vi "Actor Core.vi"(8 "error in":errorcluster, 11 "Fluke Hydra 2625A in":refnum<class "Fluke Hydra 2625A.lvclass">) -> (0 "error out":errorcluster, 3 "Actor out":refnum<class "Actor.lvclass">)   [LabVIEW 2014, in "Generic Data Acquisition.lvlib" / "Fluke Hydra.lvlib" / "Fluke Hydra 2625A.lvclass"]
doc: "(<B>Filename</B>: Actor Framework.lvlib:Actor.lvclass:Actor Core.vi)\n\nReceives messages to the actor, reacts to them, and initiates any error handling that may shut the actor down.\n\nDescendant classes may override this VI to append parallel tasks for the actor to complete while it handles messages. Overrides use the Call Parent Method node."
uses:
  Fluke Hydra 2625A.lvclass
  <vilib>/ActorFramework/Actor/Actor.lvclass
  <vilib>/ActorFramework/Actor/Actor.lvclass/Actor.ctl
  <vilib>/ActorFramework/Message Enqueuer/Message Enqueuer.lvclass/Message Enqueuer.ctl
  Display Panel/Display Panel V3 Messages/Write signal from control Msg/Write signal from control Msg.lvclass/Write signal from control Msg.ctl
  <vilib>/ActorFramework/Stop Msg/Stop Msg.lvclass/Stop Msg.ctl
  <vilib>/ActorFramework/Message Enqueuer/Init from Existing Queue.vi
  <vilib>/ActorFramework/Message Enqueuer/Enqueue.vi
  <vilib>/ActorFramework/Message Enqueuer/Enqueue Critical.vi
  <vilib>/ActorFramework/Message Priority Queue/Priority Enqueue.vi
  <vilib>/ActorFramework/Message Enqueuer/Message Enqueuer.lvclass
  Display Panel/Display Panel V3 Messages/Write signal from control Msg/Write signal from control Msg.lvclass
  Generic Data Acquisition Messages/Measure Msg/Measure Msg.lvclass
  <vilib>/ActorFramework/Stop Msg/Stop Msg.lvclass
  Generic Data Acquisition.lvclass
  Data Logger/Data Logger.lvclass
panel:
  out "i":i32
  out "Channel Names":string[](array[string])
  out "Channel Functions":i8[](array[numeric])
  out "Channel List":i8[](array[numeric])
  out "outside i":i32
  in  "Array":dbl[](array[numeric])=[0.0, 0.0]
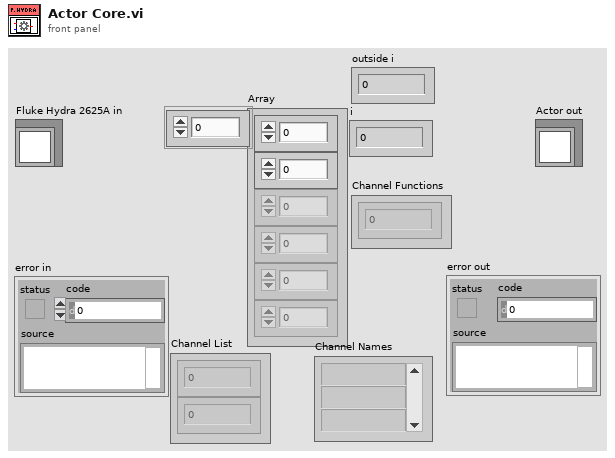
[diagram p1: front panel]
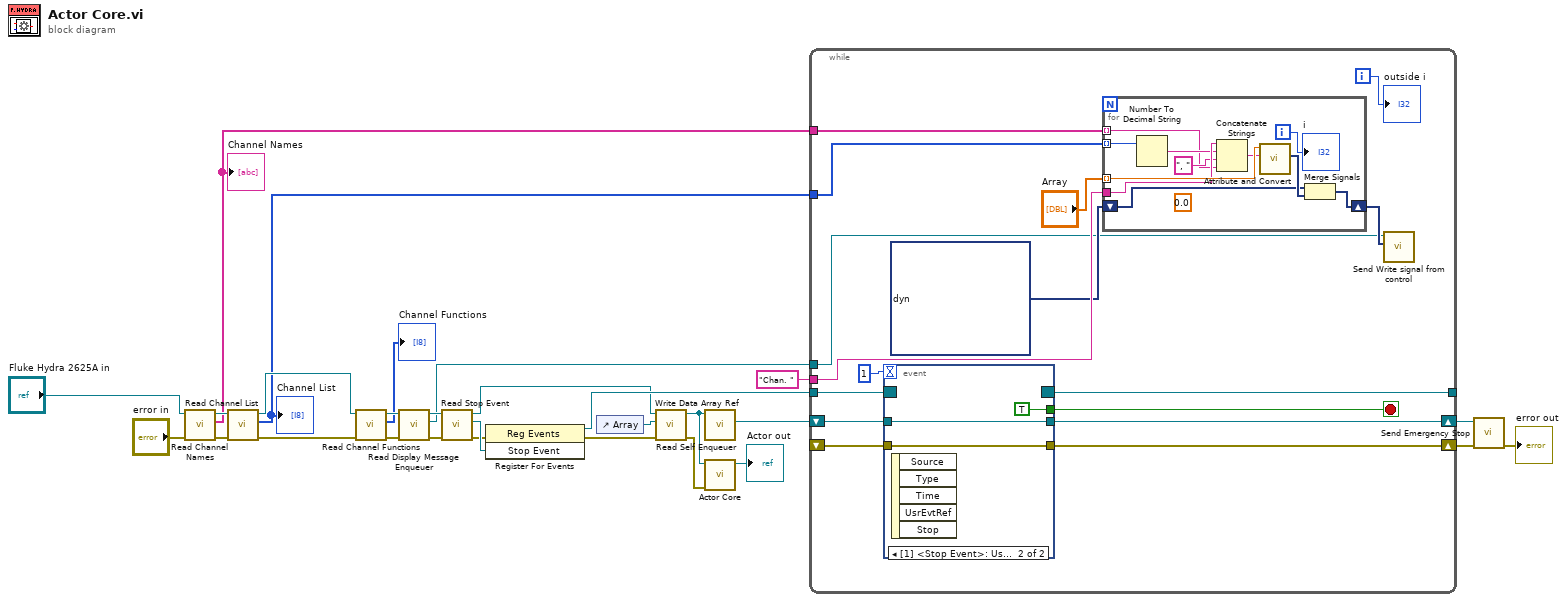
[diagram p0: block diagram]
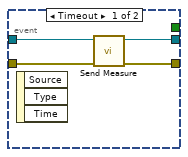
[diagram p2: hidden frame]
diagram:
  n1 = call-dynamic "Read Channel Names.vi"("error in (no error)"="error in", "Generic Data Acquisition in"="Fluke Hydra 2625A in") -> ("error out"=w4:errorcluster, "Channel Names"=w1:string[], "Generic Data Acquisition out"=w6:refnum<class "Fluke Hydra 2625A.lvclass">)  [unwired: 7 in]
  "Channel Names" <- w1
  n2 = call-dynamic "Read Channel List.vi"("error in (no error)"=w4, "Generic Data Acquisition in"=w6) -> ("error out"=w13:errorcluster, "Channel List"=w3:i8[], "Generic Data Acquisition out"=w14:refnum<class "Fluke Hydra 2625A.lvclass">)  [unwired: 7 in]
  "Channel List" <- w3
  n3 = call-dynamic "Read Channel Functions.vi"("error in (no error)"=w13, "Generic Data Acquisition in"=w14) -> ("error out"=w11:errorcluster, "Channel Functions"=→"Channel Functions":i8[], "Generic Data Acquisition out"=w12:refnum<class "Fluke Hydra 2625A.lvclass">)  [unwired: 7 in]
  n4 = call-dynamic "Read Display Message Enqueuer.vi"("error in (no error)"=w11, "Generic Instrument in"=w12) -> ("error out"=w16:errorcluster, "Actor Framework.lvlib:Message Enqueuer"=w15:refnum<class "Message Enqueuer.lvclass">, "Generic Instrument out"=w17:refnum<class "Fluke Hydra 2625A.lvclass">)  [unwired: 7 in]
  n5 = call-dynamic "Read Stop Event.vi"("error in (no error)"=w16, "Generic Instrument in"=w17) -> ("error out"=w22:errorcluster, "Stop Event"=w23:refnum<user-event>, "Generic Instrument out"=w24:refnum<class "Fluke Hydra 2625A.lvclass">)  [unwired: 7 in]
  n6 = register-events(error in=w22, w23) -> (reference out=w27:refnum<event-registration>, error out=w21:errorcluster)  [unwired: 1 in]
  n7 = control-ref of="Array"() -> (w25:refnum<vi>)
  n8 = call-dynamic "Write Data Array Ref.vi"("error in (no error)"=w21, "Data Array Ref"=w25, "Generic Instrument in"=w24) -> ("error out"=w8:errorcluster, "Generic Instrument out"=w9:refnum<class "Fluke Hydra 2625A.lvclass">)  [unwired: 7 in]
  n9 = call <vilib>:"Read Self Enqueuer.vi"("Actor"=w9) -> ("Self Enqueuer"=w26:refnum<class "Message Enqueuer.lvclass">)  [unwired: 10 in]
  n10 = call-parent "Actor Core.vi"("error in"=w8, "Actor in"=w9) -> ("Actor out"=→"Actor out":refnum<class "Actor.lvclass">)  [unwired: 8 in, 1 out]
  n11 = while {
    tunnel: w27 -> [w43]
    tunnel: [w42] -> _
    shift-right: [w40] -> w20
    shift-left: _ -> [w38]
    shift-right: [w36] -> w19
    shift-left: w26 -> [w41]
    tunnel: w15 -> [w29]
    tunnel: w3 -> [w34]
    tunnel: "Chan. " -> [w33]
    tunnel: w1 -> [w32]
    i -> [w39]
    stop <- w37 stop-if-true
    n12 = event shown="[1] <Stop Event>: User Event" {
      selector: w43 -> [_ _]
      dyn-events: [_ _] -> w42
      timeout: 1 -> [_ _]
      tunnel: [_ TRUE ("Stop Button")] -> w37
      tunnel: w41 -> [w59 w61]
      tunnel: [w58 w60] -> w40
      tunnel: w38 -> [w57 w60]
      tunnel: [w56 w61] -> w36
      event Timeout {
        n13 = event-data() -> ()  [unwired: 1 in, 3 out]
        n14 = call "Send Measure.vi"("error in (no error)"=w57, "Message Enqueuer"=w59) -> ("error out"=w58:errorcluster, "Message Enqueuer out"=w56:refnum<class "Message Enqueuer.lvclass">)  [unwired: 8 in]
      }
      event User Event {
        n15 = event-data() -> ()  [unwired: 1 in, 5 out]
      }
    }
    n16 = for {
      tunnel: "Array" -> [w55] mode=indexing
      tunnel: w34 -> [w52] mode=indexing
      tunnel: w33 -> [w54]
      tunnel: w32 -> [w50] mode=indexing
      shift-right: [w48] -> w30
      shift-left: dynamicdata [] ("Dynamic Signal Out") -> [w47]
      i -> [w45]
      (unwired) 0.0 ("Dynamic Signal Out")
      n17 = Number To Decimal String(number=w52) -> (decimal integer string=w53:string)  [unwired: 1 in]
      n18 = Concatenate Strings(w54, w53, ", " ("string"), w50) -> (w46:string)
      n19 = call "Attribute and Convert.vi"("Signal Name"=w46, "Number in"=w55) -> ("Dynamic Signal Out"=w49:dynamicdata)  [unwired: 9 in]
      n20 = Merge Signals(w47, w49) -> (w48:dynamicdata)
      "i" <- w45
    }
    n21 = call "Send Write signal from control.vi"("Waveform Chart In"=w30, "Message Enqueuer"=w29) -> ()  [unwired: 8 in, 2 out]
    "outside i" <- w39
  }
  n22 = call <vilib>:"Send Emergency Stop.vi"("error in (no error)"=w20, "Message Enqueuer"=w19) -> ("error out"=→"error out":errorcluster)  [unwired: 9 in]
